vi "Control Panel.vi"(9 "Control Panel Solenoid Up":bool, 11 "Control Panel Spin":dbl) -> ()   [LabVIEW 2019]
uses:
  <vilib>/Rock Robotics/WPI/ThirdParty/Phoenix-LabVIEW/Motor Controller/Controls/CTRE_Phoenix_MotorControl_ControlMode.ctl
  <vilib>/Rock Robotics/WPI/Solenoid/WPI_SolenoidValue.ctl
  <vilib>/Rock Robotics/WPI/Solenoid/WPI_SolenoidSetEnum.vi
panel:
  in  "Control Panel":T1 items=["PercentOutput"=0, "Position"=1, "Velocity"=2, "Current"=3, "Follower"=5, "MotionProfile"=6, "MotionMagic"=7, "MotionProfileArc"=10, "Disabled"=15]
  in  "Control Panel":T1 items=["PercentOutput"=0, "Position"=1, "Velocity"=2, "Current"=3, "Follower"=5, "MotionProfile"=6, "MotionMagic"=7, "MotionProfileArc"=10, "Disabled"=15]
  in  "Control Panel":T1 items=["PercentOutput"=0, "Position"=1, "Velocity"=2, "Current"=3, "Follower"=5, "MotionProfile"=6, "MotionMagic"=7, "MotionProfileArc"=10, "Disabled"=15]
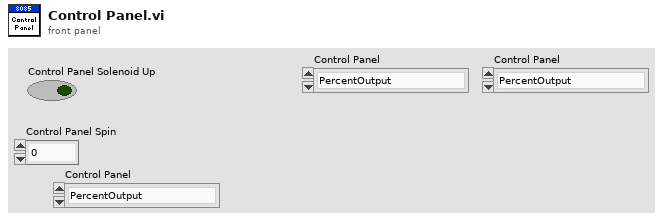
[diagram p1: front panel]
types:
  T1 = typedef "CTRE_Phoenix_MotorControl_ControlMode.ctl" = u16
  T2 = typedef "WPI_SolenoidValue.ctl" = enum16{"Off", "On", "Forward", "Reverse"}
  T3 = typedef "WPI_MotorControlDeviceRef.ctl" = cluster{"DeviceStatus":errorcluster, "Type":T4, "PWM":cluster{"PWM Channel":T5, "DeadBand":T6}, "CAN":cluster{"Device Number":u8, "SetOutput VI Ref":variant, "GetOutput VI Ref":variant, "Enable VI Ref":variant, "Disable VI Ref":variant, "Data":variant}, "Invert":bool, "DIO PWM":cluster{"PWM \"Enable\" Channel":T5, "DIOChannel":T7, "PWM Rate":dbl}}
  T4 = typedef "WPI_MotorControlType.ctl" = enum16{"PWM", "CAN", "DIO PWM"}
  T5 = typedef "FPGA_DIOPWMChannel.ctl" = enum8{"PWM 0", "PWM 1", "PWM 2", "PWM 3", "PWM 4", "PWM 5", "PWM 6", "PWM 7", "PWM 8", "PWM 9", "PWM MXP 0", "PWM MXP 1", "PWM MXP 2", "PWM MXP 3", "PWM MXP 4", "PWM MXP 5", "PWM MXP 6", "PWM MXP 7", "PWM MXP 8", "PWM MXP 9", "Invalid"}
  T6 = typedef "WPI_PWMDeadband.ctl" = cluster{"Name":string, "maxPositivePwm":i32, "minPositivePwm":i32, "centerPwm":i32, "maxNegativePwm":i32, "minNegativePwm":i32, "angularRange":u16}
  T7 = typedef "FPGA_DIOChannel.ctl" = enum8{"DIO 0", "DIO 1", "DIO 2", "DIO 3", "DIO 4", "DIO 5", "DIO 6", "DIO 7", "DIO 8", "DIO 9", "DIO MXP 0", "DIO MXP 1", "DIO MXP 2", "DIO MXP 3", "DIO MXP 4", "DIO MXP 5", "DIO MXP 6", "DIO MXP 7", "DIO MXP 8", "DIO MXP 9", "DIO MXP 10", "DIO MXP 11", "DIO MXP 12", "DIO MXP 13", "DIO MXP 14", "DIO MXP 15", "SPI Port CS1", "SPI Port CS2", "SPI Port CS3", "SPI Port MISO", "SPI Port MOSI", "Invalid"}
  T8 = typedef "WPI_SolenoidDevRef.ctl" = cluster{"DevStatus":errorcluster, "Pneumatics Control Module":u8, "Forward Solenoid Channel":T9, "Reverse Solenoid Channel":T9}
  T9 = typedef "WPI_SolenoidChannel.ctl" = enum8{"Solenoid 0", "Solenoid 1", "Solenoid 2", "Solenoid 3", "Solenoid 4", "Solenoid 5", "Solenoid 6", "Solenoid 7", "Invalid"}
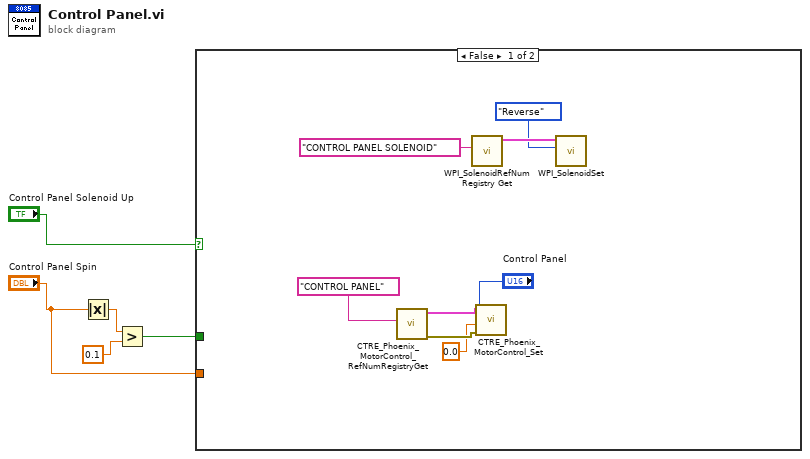
[diagram p0: block diagram]
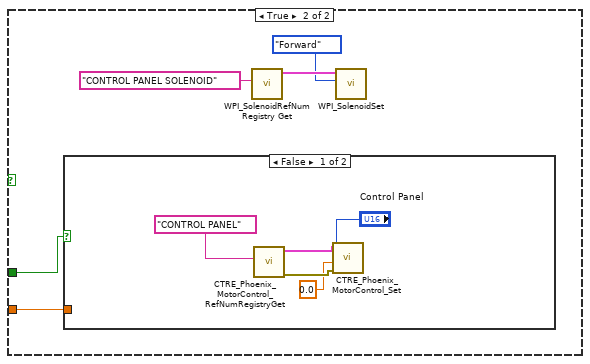
[diagram p2: hidden frame]
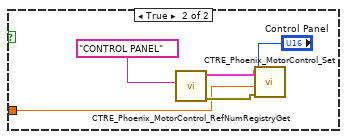
[diagram p3: hidden frame]
diagram:
  n1 = Absolute Value(x="Control Panel Spin") -> (abs(x)=w4:dbl)
  n2 = Greater?(x=w4, y=0.1) -> (0:w2:bool)
  n3 = case shown="False" "Control Panel Solenoid Up" {
    tunnel: w2 -> [_ w15]
    tunnel: "Control Panel Spin" -> [_ w14]
    frame False {
      n4 = call <vilib>:"CTRE_Phoenix_MotorControl_RefNumRegistryGet.vi"("refnum name"="CONTROL PANEL") -> ("error out"=w9:errorcluster, "PhoenixMotorControlDevRef"=w10:T3)  [unwired: 9 in]
      n5 = call <vilib>:"WPI_SolenoidRefNum Registry Get.vi"("refnum name"="CONTROL PANEL SOLENOID") -> ("SolenoidDevRef"=w13:T8)  [unwired: 9 in, 1 out]
      n6 = call <vilib>:"CTRE_Phoenix_MotorControl_Set.vi"("error in (no error)"=w9, "Output"=0.0, "Control Mode"="Control Panel", "PhoenixMotorControlDevRef"=w10) -> ()  [unwired: 6 in, 2 out]
      n7 = call-poly <vilib>:"WPI_SolenoidSet.vi"("Value"=WPI_SolenoidValue."Reverse", "SolenoidDevRef"=w13) -> ()  [unwired: 8 in, 2 out]
    }
    frame True {
      n8 = case shown="False" w15 {
        tunnel: w14 -> [_ w24]
        frame False {
          n9 = call <vilib>:"CTRE_Phoenix_MotorControl_RefNumRegistryGet.vi"("refnum name"="CONTROL PANEL") -> ("error out"=w22:errorcluster, "PhoenixMotorControlDevRef"=w23:T3)  [unwired: 9 in]
          n10 = call <vilib>:"CTRE_Phoenix_MotorControl_Set.vi"("error in (no error)"=w22, "Output"=0.0, "Control Mode"="Control Panel", "PhoenixMotorControlDevRef"=w23) -> ()  [unwired: 6 in, 2 out]
        }
        frame True {
          n11 = call <vilib>:"CTRE_Phoenix_MotorControl_RefNumRegistryGet.vi"("refnum name"="CONTROL PANEL") -> ("error out"=w27:errorcluster, "PhoenixMotorControlDevRef"=w28:T3)  [unwired: 9 in]
          n12 = call <vilib>:"CTRE_Phoenix_MotorControl_Set.vi"("error in (no error)"=w27, "Output"=w24, "Control Mode"="Control Panel", "PhoenixMotorControlDevRef"=w28) -> ()  [unwired: 6 in, 2 out]
        }
      }
      n13 = call <vilib>:"WPI_SolenoidRefNum Registry Get.vi"("refnum name"="CONTROL PANEL SOLENOID") -> ("SolenoidDevRef"=w18:T8)  [unwired: 9 in, 1 out]
      n14 = call-poly <vilib>:"WPI_SolenoidSet.vi"("Value"=WPI_SolenoidValue."Forward", "SolenoidDevRef"=w18) -> ()  [unwired: 8 in, 2 out]
    }
  }
